vi "Power Measurement Error Code List Mode.vi"(6 "Detector Type (RMS)":i32(ring) items=["RMS", "Minimum", "Maximum"], 7 "Result Type (Current)":i32(ring) items=["Current", "Average", "Peak"], 8 "error in (no error)":errorcluster, 9 "Step Index (1)":i32=1, 10 "Instance (1)":i32=1, 11 "VISA resource name":refnum<visa-resource-name>) -> (0 "error out":errorcluster, 2 "Error Code":i32, 3 "VISA resource name out":refnum<visa-resource-name>)   [LabVIEW 2015, in "Rohde&Schwarz CMXP GPRF.lvlib"]
doc: "Returns a single-value error code for each result.\n\nAttribute:\n-\n\nRemote-control commands:\nCALCulate:GPRF:MEAS<i>:POWer:LIST:CURRent?\nCALCulate:GPRF:MEAS<i>:POWer:LIST:MAXimum:CURRent?\nCALCulate:GPRF:MEAS<i>:POWer:LIST:MINimum:CURRent?\nCALCulate:GPRF:MEAS<i>:POWer:LIST:AVERage?\nCALCulate:GPRF:MEAS<i>:POWer:LIST:PEAK:MAXimum?\nCALCulate:GPRF:MEAS<i>:POWer:LIST:PEAK:MINimum?"
uses:
  <instrlib>/Rohde&Schwarz CMXP GPRF/Rohde&Schwarz CMXP GPRF.lvlib
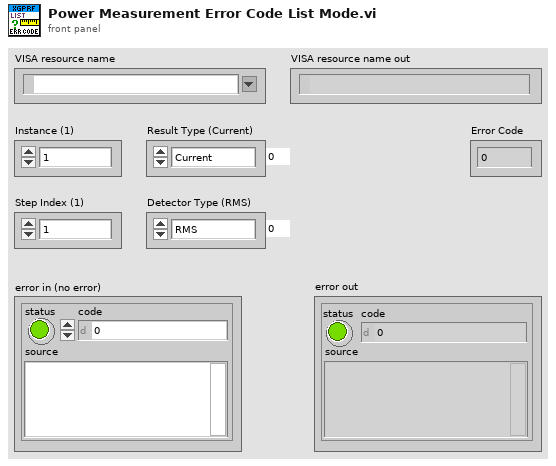
[diagram p1: front panel]
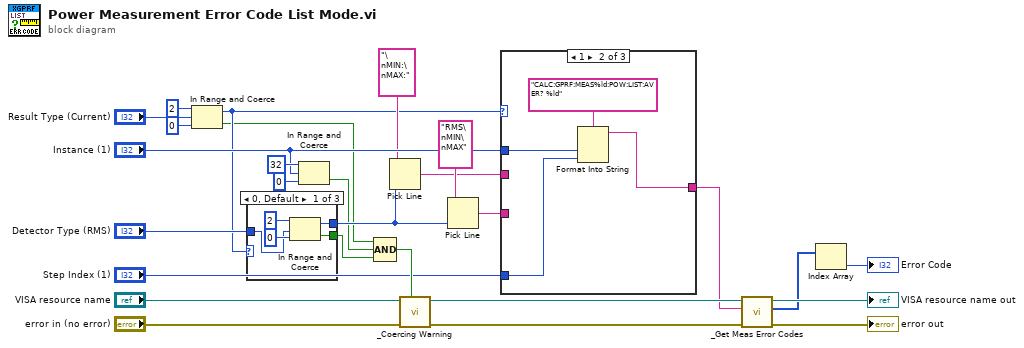
[diagram p0: block diagram]
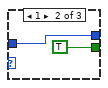
[diagram p2: hidden frame]
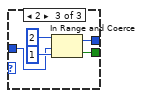
[diagram p3: hidden frame]
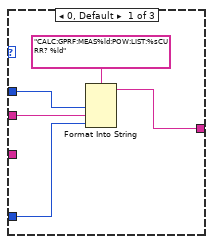
[diagram p4: hidden frame]
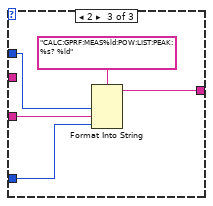
[diagram p5: hidden frame]
diagram:
  n1 = In Range and Coerce(upper limit=2, x="Result Type (Current)", lower limit=0) -> (coerced(x)=w5:i32, In Range?=w2:bool)
  n2 = case shown="0, Default" w5 {
    tunnel: [w30 TRUE w37] -> w4
    tunnel: [w29 w33 w36] -> w21
    tunnel: "Detector Type (RMS)" -> [w28 w33 w35]
    frame 0, Default {
      n3 = In Range and Coerce(upper limit=2, x=w28, lower limit=0) -> (coerced(x)=w29:i32, In Range?=w30:bool)
    }
    frame 1 {
    }
    frame 2 {
      n4 = In Range and Coerce(upper limit=2, x=w35, lower limit=1) -> (coerced(x)=w36:i32, In Range?=w37:bool)
    }
  }
  n5 = In Range and Coerce(upper limit=32, x="Instance (1)", lower limit=0) -> (In Range?=w3:bool)  [unwired: 1 out]
  n6 = Compound Arithmetic op=AND(w2, w3, w4) -> (w25:bool)
  n7 = Pick Line(multi-line string="\nMIN:\nMAX:", line index=w21) -> (output string=w20:string)  [unwired: 1 in]
  n8 = call <instrlib>:"_Coercing Warning.vi"("In Range?"=w25, "error in (no error)"="error in (no error)", "VISA resource name"="VISA resource name") -> ("error out"=w15:errorcluster, "VISA resource name out"=w16:refnum<visa-resource-name>)  [unwired: 7 in]
  n9 = Pick Line(multi-line string="RMS\nMIN\nMAX", line index=w21) -> (output string=w19:string)  [unwired: 1 in]
  n10 = case shown="1" w5 {
    tunnel: "Instance (1)" -> [w41 w47 w50]
    tunnel: [w43 w46 w52] -> w1
    tunnel: "Step Index (1)" -> [w40 w45 w49]
    tunnel: w20 -> [w42 _ _]
    tunnel: w19 -> [_ _ w51]
    frame 0, Default {
      n11 = Format Into String(format string="CALC:GPRF:MEAS%ld:POW:LIST:%sCURR? %ld", w41, w42, w40) -> (resulting string=w43:string)  [unwired: 2 in, 1 out]
    }
    frame 1 {
      n12 = Format Into String(format string="CALC:GPRF:MEAS%ld:POW:LIST:AVER? %ld", w47, w45) -> (resulting string=w46:string)  [unwired: 2 in, 1 out]
    }
    frame 2 {
      n13 = Format Into String(format string="CALC:GPRF:MEAS%ld:POW:LIST:PEAK:%s? %ld", w50, w51, w49) -> (resulting string=w52:string)  [unwired: 2 in, 1 out]
    }
  }
  n14 = call <instrlib>:"_Get Meas Error Codes.vi"("error in (no error)"=w15, "Command"=w1, "VISA resource name"=w16) -> ("error out"=→"error out":errorcluster, "Error Codes"=w12:i32[], "VISA resource name out"=→"VISA resource name out":refnum<visa-resource-name>)  [unwired: 5 in, 1 out]
  n15 = Index Array(array=w12) -> (element=→"Error Code":i32)  [unwired: 1 in]
